vi "PicoScope4000ExampleAdvancedTrigger.vi"() -> ()   [LabVIEW 2012]
doc: "This example demonstrates how to use the PicoScope Labview library to collect data using block mode."
uses:
  shared/PicoBuffers.ctl
  shared/Acquisition Settings.ctl
  PicoScope4000Lib/PicoScope4000AnalogChannelSettingsIEPE.ctl
  PicoScope4000Lib/PicoScope4000Buffer and Transfer Settings.ctl
panel:
  in  "Pulse Width Qualifier Conditions":T1 {"Aux" items=["Don't Care", "True", "False"]; "Ext" items=["Don't Care", "True", "False"]; "Channel D" items=["Don't Care", "True", "False"]; "Channel C" items=["Don't Care", "True", "False"]; "Channel B" items=["Don't Care", "True", "False"]; "Channel A" items=["Don't Care", "True", "False"]; "Condition Logic" items=["AND", "OR", "XOR"]}
  in  "Trigger Conditions":T2 {"Aux" items=["Don't Care", "True", "False"]; "Pulse Width Qualifier" items=["Don't Care", "True", "False"]; "Ext" items=["Don't Care", "True", "False"]; "Channel D" items=["Don't Care", "True", "False"]; "Channel C" items=["Don't Care", "True", "False"]; "Channel B" items=["Don't Care", "True", "False"]; "Channel A" items=["Don't Care", "True", "False"]; "Condition Logic" items=["AND", "OR", "XOR"]}
  in  "Auto Trigger (ms)":i32=1000
  in  "Pulse Width Qualifier Settings":T3={"Direction"=2, "Lower Limit"=0, "Upper Limit"=0, "Pulse Width Type"=1} {"Pulse Width Type" items=["None", "Less Than", "Greater Than", "In Range", "Out of Range"]; "Direction" items=["Rising"=2, "Falling"=3, "Rising Lower"=7, "Above"=0, "Below"=1, "Rising or Falling"=4, "Falling Lower"=8, "Below Lower"=6, "Above Lower"=5]}
  in  "Channel Trigger Properties":T4={"Channel A Trigger Properties"={"thresholdUpper"=0, "thresholdUpperHysteresis"=0, "thresholdLower"=0, "thresholdLowerHysteresis"=0, "Threshold Mode"=0, "Direction"=2, "Available"=TRUE}, "Channel B Trigger Properties"={"thresholdUpper"=0, "thresholdUpperHysteresis"=0, "thresholdLower"=0, "thresholdLowerHysteresis"=0, "Threshold Mode"=0, "Direction"=2, "Available"=FALSE}, "Channel C Trigger Properties"={"thresholdUpper"=0, "thresholdUpperHysteresis"=0, "thresholdLower"=0, "thresholdLowerHysteresis"=0, "Threshold Mode"=0, "Direction"=2, "Available"=FALSE}, "Channel D Trigger Properties"={"thresholdUpper"=0, "thresholdUpperHysteresis"=0, "thresholdLower"=0, "thresholdLowerHysteresis"=0, "Threshold Mode"=0, "Direction"=2, "Available"=FALSE}} {"Channel D Trigger Properties"."Direction" items=["Above / Inside", "Below / Outside", "Rising / Enter", "Falling / Exit", "Rising or Falling / Enter or Exit", "Above Lower", "Below Lower", "Rising Lower", "Falling Lower", "Positive Runt", "Negative Runt"]; "Channel D Trigger Properties"."Threshold Mode" items=["Level", "Window"]; "Channel C Trigger Properties"."Direction" items=["Above / Inside", "Below / Outside", "Rising / Enter", "Falling / Exit", "Rising or Falling / Enter or Exit", "Above Lower", "Below Lower", "Rising Lower", "Falling Lower", "Positive Runt", "Negative Runt"]; "Channel C Trigger Properties"."Threshold Mode" items=["Level", "Window"]; "Channel B Trigger Properties"."Direction" items=["Above / Inside", "Below / Outside", "Rising / Enter", "Falling / Exit", "Rising or Falling / Enter or Exit", "Above Lower", "Below Lower", "Rising Lower", "Falling Lower", "Positive Runt", "Negative Runt"]; "Channel B Trigger Properties"."Threshold Mode" items=["Level", "Window"]; "Channel A Trigger Properties"."Direction" items=["Above / Inside", "Below / Outside", "Rising / Enter", "Falling / Exit", "Rising or Falling / Enter or Exit", "Above Lower", "Below Lower", "Rising Lower", "Falling Lower", "Positive Runt", "Negative Runt"]; "Channel A Trigger Properties"."Threshold Mode" items=["Level", "Window"]}
  in  "Channel B Settings":T5={"Enabled"=FALSE, "Range"=6, "Bandwidth Limit"=0, "Coupling"=1} {"Coupling" items=["AC", "DC", "IEPE"]; "Bandwidth Limit" items=["Off", "200kHz"]; "Range" items=["10 mV", "20 mV", "50 mV", "100 mV", "200 mV", "500 mV", "1 V", "2 V", "5 V", "10 V", "20 V", "50 V ", "100 V"]}
  out "Unit Info":T6
  in  "PS4262 Ext. Trigger Range":u32(ring)=5 items=["500 mV"=5, "5 V"=8]
  in  "Channel A Settings":T5={"Enabled"=TRUE, "Range"=6, "Bandwidth Limit"=0, "Coupling"=1} {"Coupling" items=["AC", "DC", "IEPE"]; "Bandwidth Limit" items=["Off", "200kHz"]; "Range" items=["10 mV", "20 mV", "50 mV", "100 mV", "200 mV", "500 mV", "1 V", "2 V", "5 V", "10 V", "20 V", "50 V ", "100 V"]}
  out "overflow":i16 format="%08b"
  in  "Apply Settings":bool
  out "error out":errorcluster
  in  "Data file":path=path "PicoScope4000ExampleBlock ChA Data"
  in  "Buffer and Transfer Settings":T7={"startIndex"=0, "Samples"=1000000, "Down Sample Ratio"=1, "Down-Sample Mode"=0} {"Down-Sample Mode" items=["None", "Aggregate", "Average"]; "Down Sample Ratio" step=1; "Samples" format="%_6p"}
  in  "Acquisition Settings":T8={"preTriggerSamples"=0, "postTriggerSamples"=1000000, "timebase"=3} {"postTriggerSamples" format="%_6p"; "preTriggerSamples" format="%_6p"}
  out "Properties Panel":T9 {"Max Total Capture Time Available (sec)" format="%.3p"; "Sample Frequency" format="%.6p"; "Sample Rate" format="%.3p"; "Max Samples Available" format="%_6p"; "Total Capture Time (sec)" format="%.3p"}
  in  "stop":bool
  out "Analog Channels":cluster{i32, dbl, "Data":dbl[]}[](graph)
  in  "Serial Number":string
  in  "Use Serial Number":bool
  in  "error in (no error)":errorcluster
  # "Bit 0 = ChA"
  # "For Condition Logic Suggested settings;\nFor AND, XOR logic-(parallel triggers)\nUse level-type triggers (Level or Inside/outside Window Triggers)\n\nFor OR logic- (single channel)\nUse edge types (e.g. rising, falling, entering window)"
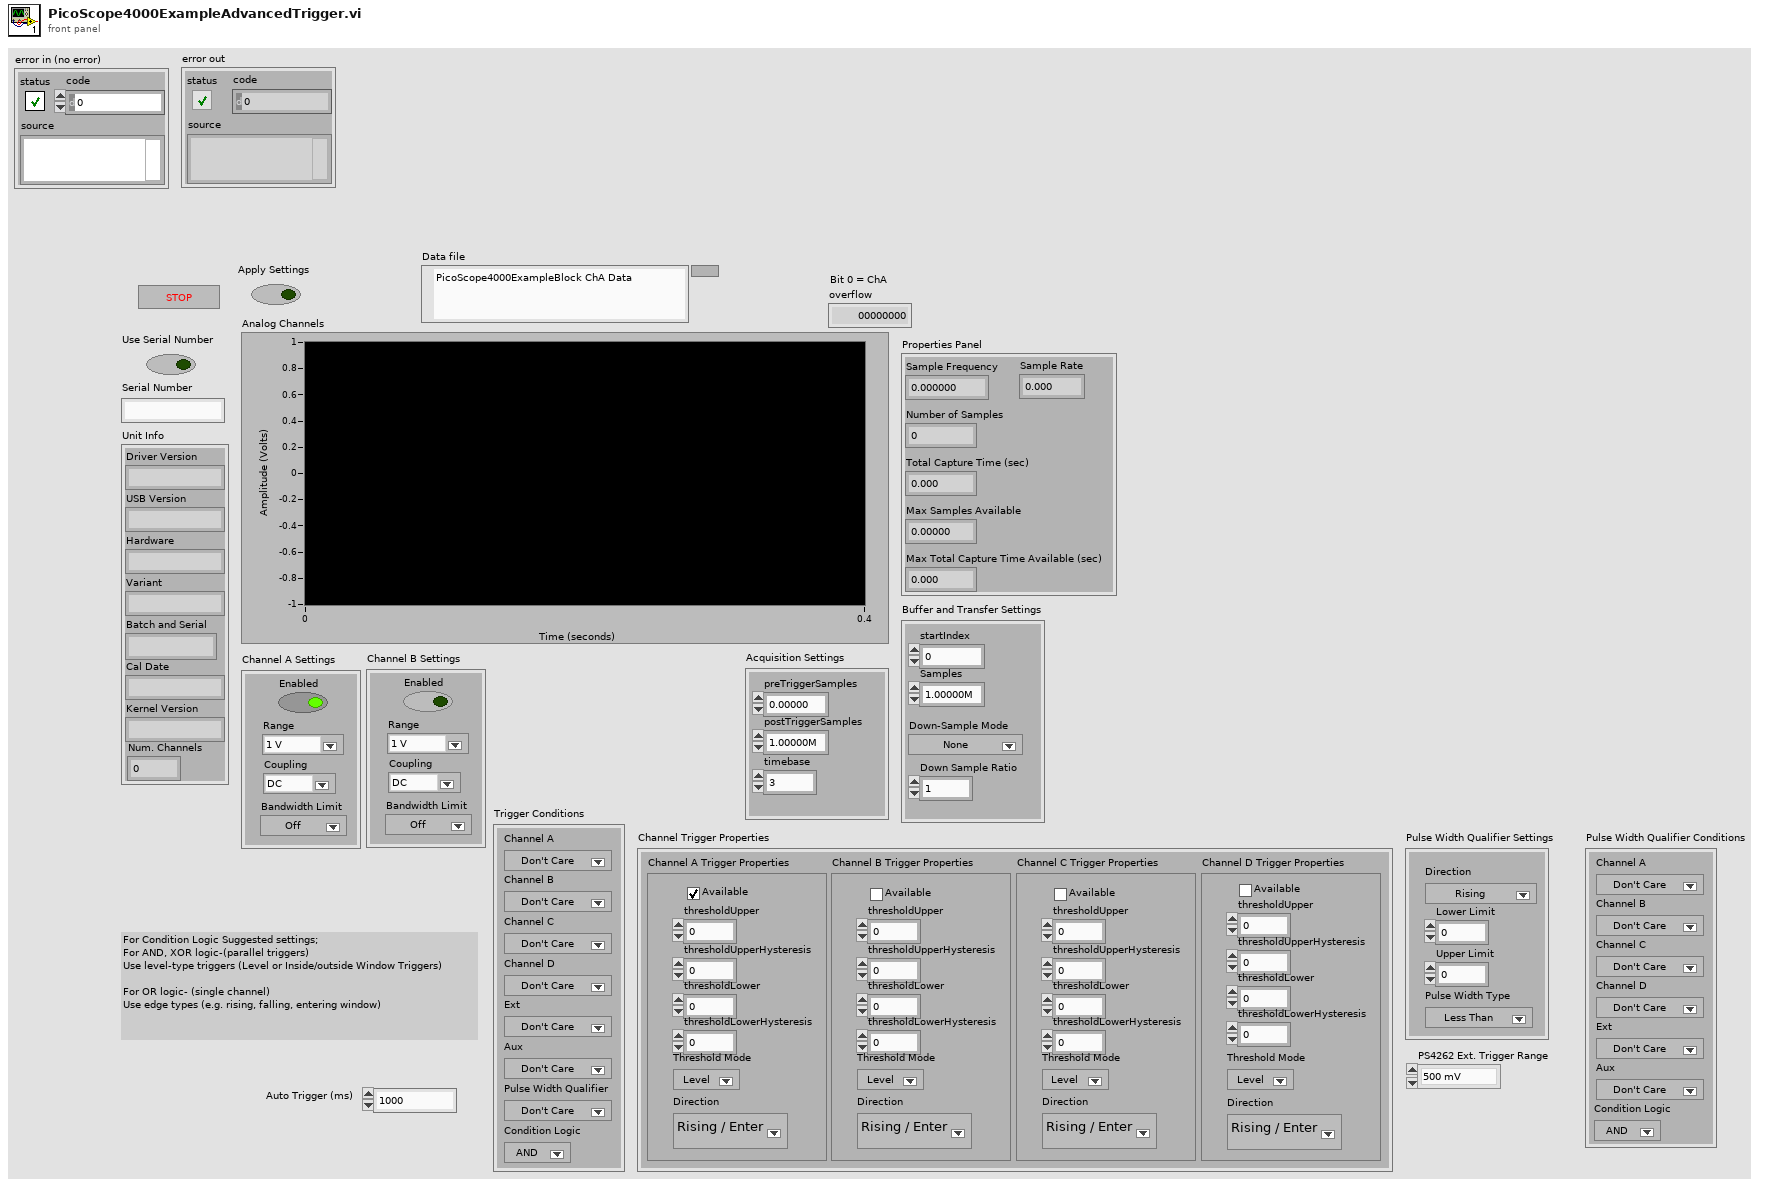
[diagram p1: front panel]
types:
  T1 = cluster{"Channel A":u16, "Channel B":u16, "Channel C":u16, "Channel D":u16, "Ext":u16, "Aux":u16, "Condition Logic":u16}
  T2 = cluster{"Channel A":u16, "Channel B":u16, "Channel C":u16, "Channel D":u16, "Ext":u16, "Aux":u16, "Pulse Width Qualifier":u16, "Condition Logic":u16}
  T3 = cluster{"Direction":u32, "Lower Limit":u32, "Upper Limit":u32, "Pulse Width Type":u32}
  T4 = cluster{"Channel A Trigger Properties":cluster{"thresholdUpper":i16, "thresholdUpperHysteresis":u16, "thresholdLower":i16, "thresholdLowerHysteresis":u16, "Threshold Mode":i32, "Direction":u32, "Available":bool}, "Channel B Trigger Properties":cluster{"thresholdUpper":i16, "thresholdUpperHysteresis":u16, "thresholdLower":i16, "thresholdLowerHysteresis":u16, "Threshold Mode":i32, "Direction":u32, "Available":bool}, "Channel C Trigger Properties":cluster{"thresholdUpper":i16, "thresholdUpperHysteresis":u16, "thresholdLower":i16, "thresholdLowerHysteresis":u16, "Threshold Mode":i32, "Direction":u32, "Available":bool}, "Channel D Trigger Properties":cluster{"thresholdUpper":i16, "thresholdUpperHysteresis":u16, "thresholdLower":i16, "thresholdLowerHysteresis":u16, "Threshold Mode":i32, "Direction":u32, "Available":bool}}
  T5 = typedef "PicoScope4000AnalogChannelSettingsIEPE.ctl" = cluster{"Enabled":bool, "Range":u16, "Bandwidth Limit":i16, "Coupling":u16}
  T6 = cluster{"Driver Version":string, "USB Version":string, "Hardware":string, "Variant":string, "Batch and Serial":string, "Cal Date":string, "Kernel Version":string, "Num. Channels":i16}
  T7 = typedef "PicoScope4000Buffer and Transfer Settings.ctl" = cluster{"startIndex":u64, "Samples":u64, "Down Sample Ratio":u64, "Down-Sample Mode":u32}
  T8 = typedef "Acquisition Settings.ctl" = cluster{"preTriggerSamples":u64, "postTriggerSamples":u64, "timebase":u32}
  T9 = cluster{"Sample Frequency":dbl, "Sample Rate":dbl, "Max Samples Available":u64, "Number of Samples":u64, "Total Capture Time (sec) ":dbl, "Max Total Capture Time Available (sec)":dbl}
  T10 = enum16{"open", "open or create", "create or replace", "create", "open (read-only)"}
  T11 = typedef "PicoBuffers.ctl" = cluster{"Max Buffer Pointers":u64[][][], "Min Buffer Pointers":u64[][][], "StreamingDataInfo":cluster{"Channel":u32, "Down-Sample Mode":u32, "PICO_DATA_TYPE":enum32{"PICO_INT8_T", "PICO_INT16_T", "PICO_INT32_T", "PICO_UINT32_T", "PICO_INT64_T", ""}, "Samples":i32, "bufferIndex":u64, "startIndex":i32, "overflow":i16}[][]}
  T12 = cluster{"Channel A Buffer":i16[], "Channel B Buffer":i16[], "Channel C Buffer":i16[], "Channel D Buffer":i16[], "Channel E Buffer":i16[], "Channel F Buffer":i16[], "Channel G Buffer":i16[], "Channel H Buffer":i16[], "Port 0 Buffer":i16[], "Port 1 Buffer":i16[]}[]
  T13 = cluster{"Channel A Buffer":i16[], "Channel B Buffer":i16[], "Channel C Buffer":i16[], "Channel D Buffer":i16[], "Channel E Buffer":i16[], "Channel F Buffer":i16[], "Channel G Buffer":i16[], "Channel H Buffer":i16[], "Port 0 Buffer":i16[], "Port 1 Buffer":i16[]}
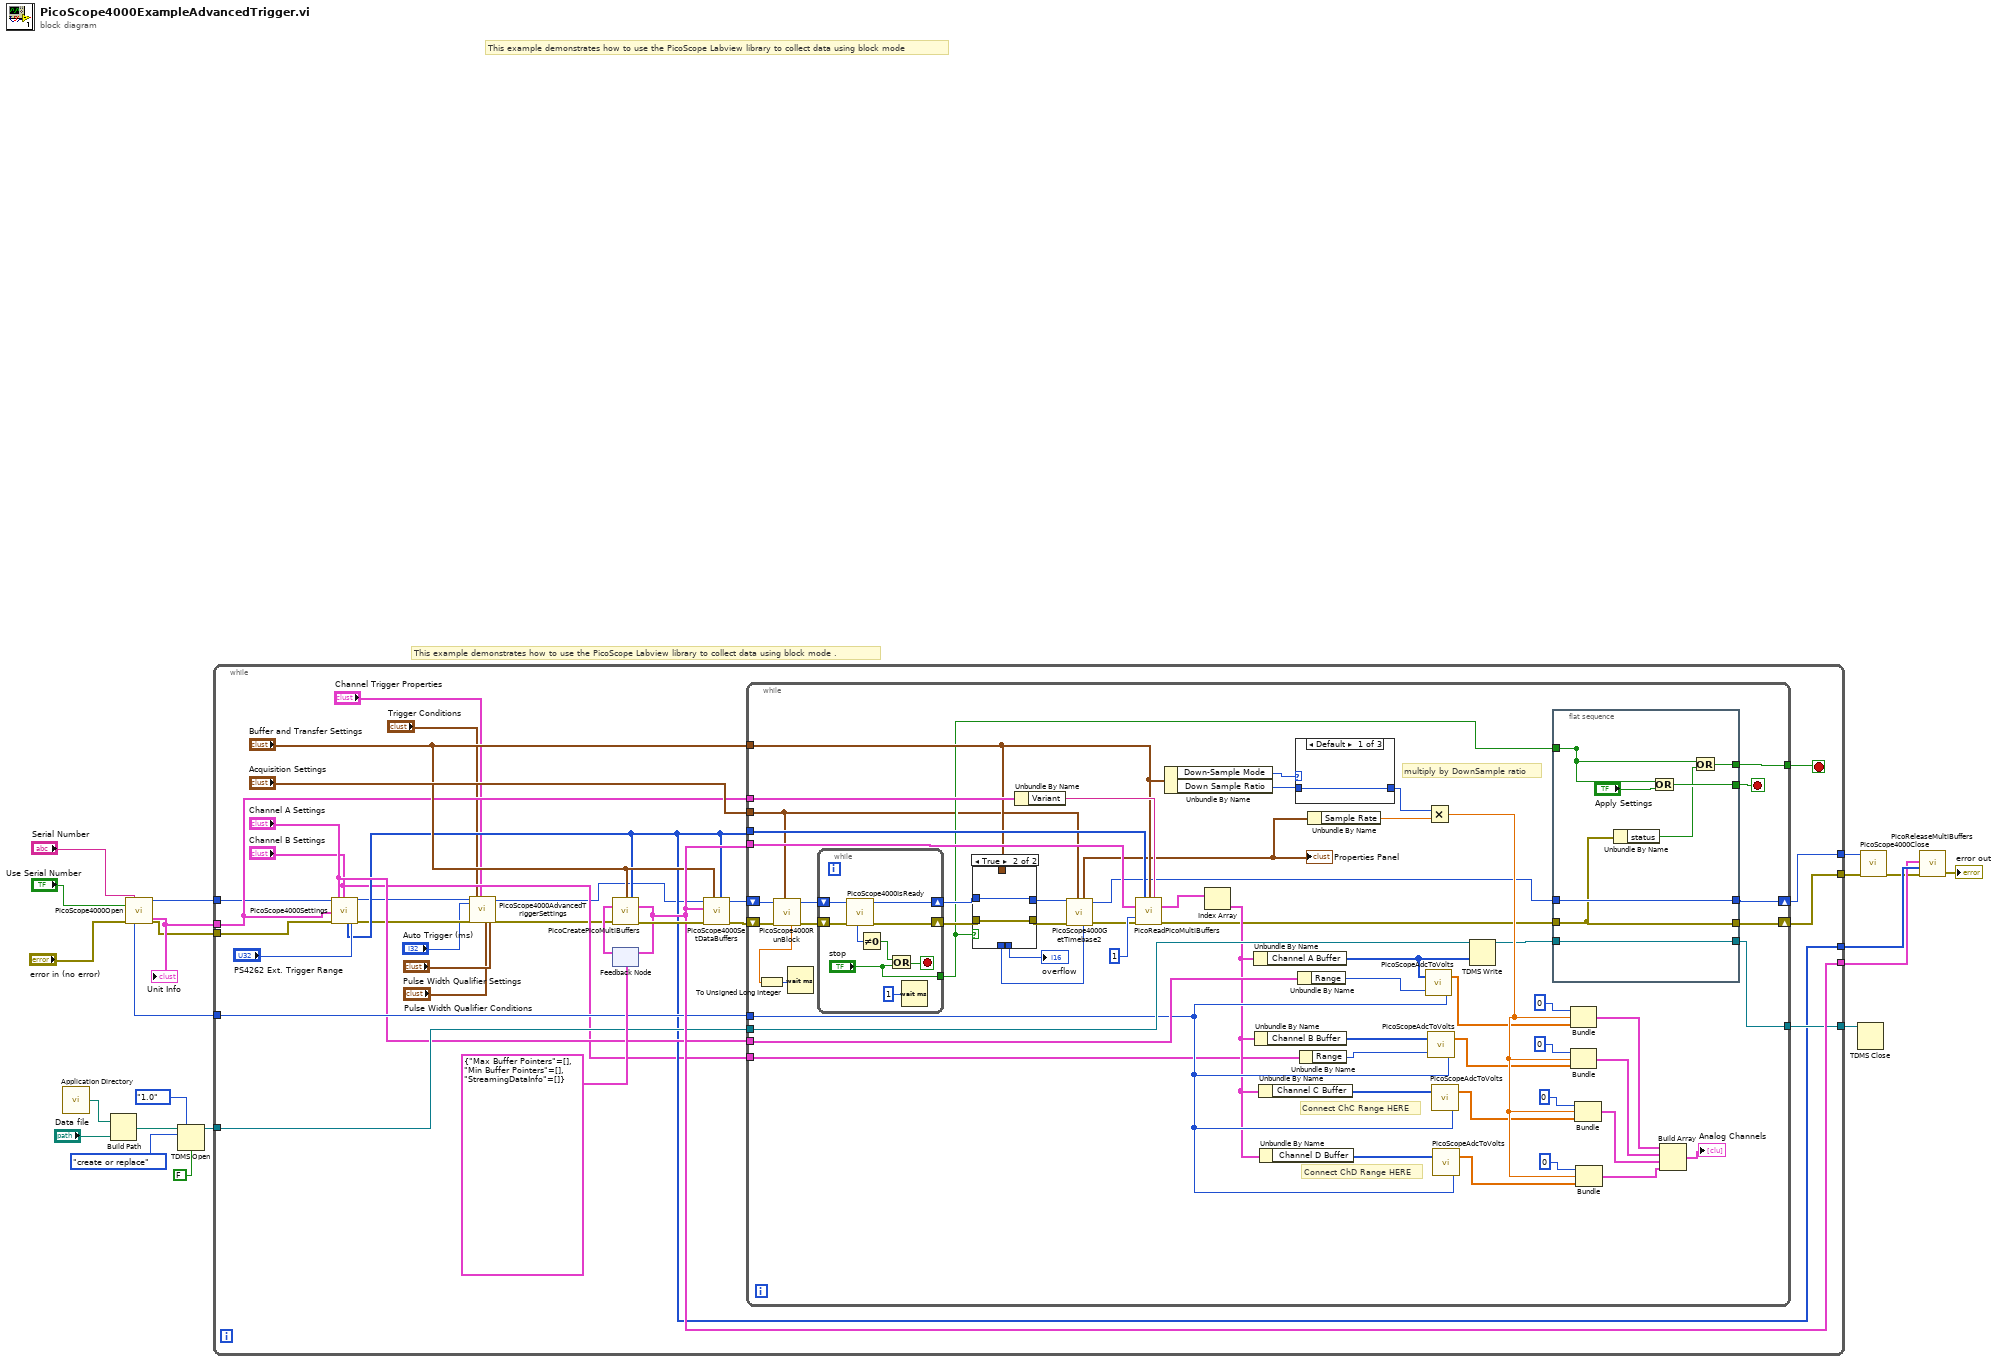
[diagram p0: block diagram]
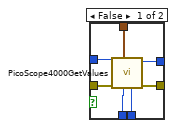
[diagram p2: hidden frame]
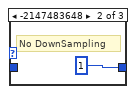
[diagram p3: hidden frame]
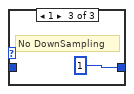
[diagram p4: hidden frame]
diagram:
  # "This example demonstrates how to use the PicoScope Labview library to collect data using block mode ."
  # "This example demonstrates how to use the PicoScope Labview library to collect data using block mode"
  n1 = call <vilib>:"Application Directory.vi"() -> ("Application Directory"=w14:path)
  n2 = Build Path(base path=w14, name or relative path="Data file") -> (appended path=w15:path)
  n3 = call "PicoScope4000Open.vi"("Serial Number"="Serial Number", "Use Serial Number"="Use Serial Number", "error in (no error)"="error in (no error)") -> ("handle"=w5:i16, "Max ADC value"=w10:i16, "Unit Info"=w6:T6, "error out"=w4:errorcluster)  [unwired: 9 in]
  "Unit Info" <- w6
  n4 = TDMS Open(6:FALSE ("disable buffering? (T)"), 7:enum16{"1.0", "2.0"}."1.0" ("file format version (2.0)"), 10:T10."create or replace" ("operation (0:open)"), 11:w15) -> (3:w12:refnum<k34>)  [unwired: 2 in, 1 out]
  n5 = while {
    tunnel: w10 -> [w45]
    tunnel: [w32] -> w21
    tunnel: [w48] -> w20
    tunnel: [w43] -> w13
    tunnel: w12 -> [w47]
    tunnel: [w44] -> w2
    tunnel: [w41] -> w9
    tunnel: w6 -> [w35]
    tunnel: w5 -> [w34]
    tunnel: w4 -> [w33]
    stop <- w42 stop-if-true
    n6 = call "PicoScope4000Settings.vi"("handle in"=w34, "Unit Info"=w35, "error in"=w33, "Channel A Settings"="Channel A Settings", "Channel B Settings"="Channel B Settings", "PicoScope 4262 Ext. Trigger Range"="PS4262 Ext. Trigger Range") -> ("Enabled array"=w32:i16[], "handle out"=w29:i16, "error out"=w30:errorcluster)  [unwired: 11 in]
    n7 = call "PicoScope4000AdvancedTriggerSettings.vi"("handle in"=w29, "error in"=w30, "Trigger Conditions"="Trigger Conditions", "Channel Trigger Properties"="Channel Trigger Properties", "Auto Trigger (ms)"="Auto Trigger (ms)", "Pulse Width Qualifier Conditions"="Pulse Width Qualifier Conditions", "Pulse Width Qualifier Settings"="Pulse Width Qualifier Settings") -> ("handle out"=w22:i16, "error out"=w23:errorcluster)  [unwired: 11 in]
    n8 = feedback #1(T11 {"Max Buffer Pointers"=[], "Min Buffer Pointers"=[], "StreamingDataInfo"=[]} ("Data Pointers")) -> (w50:T11)
    n9 = call "PicoCreatePicoMultiBuffers.vi"("Buffer and Transfer Settings"="Buffer and Transfer Settings", "enabled array"=w32, "Data Pointers In"=w50, "error in (no error)"=w23) -> ("Data Pointers"=w48:T11, "error out"=w49:errorcluster)  [unwired: 10 in]
    n10 = feedback-in #1(w48) -> ()
    n11 = call "PicoScope4000SetDataBuffers.vi"("enabled array"=w32, "Buffer and Transfer Settings"="Buffer and Transfer Settings", "error in (no error)"=w49, "Data Pointers In"=w48, "handle in"=w22) -> ("error out"=w40:errorcluster, "handle out"=w39:i16)  [unwired: 5 in]
    n12 = while {
      tunnel: w48 -> [w111]
      tunnel: "Buffer and Transfer Settings" -> [w65]
      tunnel: w32 -> [w102]
      tunnel: "Channel A Settings" -> [w101]
      tunnel: "Acquisition Settings" -> [w56]
      tunnel: w45 -> [w100]
      tunnel: w35 -> [w97]
      tunnel: [w72] -> w42
      shift-right: [w76] -> w44
      shift-left: w40 -> [w66]
      shift-right: [w70] -> w41
      shift-left: w39 -> [w67]
      tunnel: w47 -> [w110]
      tunnel: [w74] -> w43
      tunnel: "Channel B Settings" -> [w53]
      stop <- w71 stop-if-true
      # "Connect ChD Range HERE"
      # "Connect ChC Range HERE"
      # "multiply by DownSample ratio"
      n13 = call "PicoScope4000RunBlock.vi"("Acquisition Settings"=w56, "error in (no error)"=w66, "handle in"=w67) -> ("error out"=w104:errorcluster, "handle out"=w103:i16, "timeIndisposedMs"=w54:dbl)  [unwired: 5 in, 1 out]
      n14 = To Unsigned Long Integer(number=w54) -> (unsigned 32bit integer=w55:u32)
      n15 = Wait (ms)(milliseconds to wait=w55) -> ()  [unwired: 1 out]
      n16 = while {
        shift-right: [w136] -> w68
        shift-left: w104 -> [w137]
        shift-right: [w135] -> w69
        shift-left: w103 -> [w134]
        tunnel: ["stop"] -> w64
        stop <- w131 stop-if-true
        n17 = call "PicoScope4000IsReady.vi"("error in (no error)"=w137, "handle in"=w134) -> ("error out"=w136:errorcluster, "handle out"=w135:i16, "ready"=w133:i16)  [unwired: 7 in]
        n18 = Not Equal To 0?(x=w133) -> (x != 0?=w132:bool)
        n19 = Or(x=w132, y="stop") -> (x .or. y?=w131:bool)
        n20 = Wait (ms)(milliseconds to wait=u32 1) -> ()  [unwired: 1 out]
      }
      n21 = case shown="True" w64 {
        tunnel: w68 -> [w118 w119]
        tunnel: w69 -> [w117 w120]
        tunnel: [w116 w120] -> w58
        tunnel: [w115 w119] -> w59
        tunnel: w65 -> [w114 _]
        tunnel: [w113 _] -> w63
        tunnel: [w112 _] -> w62
        frame False {
          n22 = call "PicoScope4000GetValues.vi"("Buffer and Transfer Settings"=w114, "error in (no error)"=w118, "handle in"=w117) -> ("error out"=w115:errorcluster, "handle out"=w116:i16, "overflow"=w113:i16, "noOfSamples"=w112:u64)  [unwired: 5 in]
        }
        frame True {
        }
      }
      "overflow" <- w63
      n23 = Unbundle By Name(w97) -> ("Variant"=w98:string)
      n24 = call "PicoScope4000GetTimebase2.vi"("Number of Samples"=w62, "Acquisition Settings"=w56, "error in (no error)"=w59, "handle in"=w58) -> ("error out"=w60:errorcluster, "handle out"=w57:i16, "Properties Panel"=w61:T9)  [unwired: 5 in]
      "Properties Panel" <- w61
      n25 = call "PicoReadPicoMultiBuffers.vi"("enabled array"=w102, "Buffer and Transfer Settings"=w65, "Variant"=w98, "Data Pointers"=w111, "No of Buffers"=1, "error in (no error)"=w60) -> ("MultiBuffers (Max or non-aggregated)"=w109:T12, "error out"=w73:errorcluster)  [unwired: 7 in, 1 out]
      n26 = Unbundle By Name(w65) -> ("Down-Sample Mode"=w107:u32, "Down Sample Ratio"=w108:u64)
      n27 = Index Array(array=w109) -> (element=w77:T13)  [unwired: 1 in]
      n28 = Unbundle By Name(w77) -> ("Channel A Buffer"=w86:i16[])
      n29 = Unbundle By Name(w77) -> ("Channel B Buffer"=w92:i16[])
      n30 = Unbundle By Name(w77) -> ("Channel C Buffer"=w84:i16[])
      n31 = Unbundle By Name(w77) -> ("Channel D Buffer"=w80:i16[])
      n32 = case shown="Default" w107 {
        tunnel: [w138 u64 1 ("Down Sample Ratio") u64 1 ("Down Sample Ratio")] -> w105
        tunnel: w108 -> [w138 _ _]
        frame Default {
        }
        frame -2147483648 {
          # "No DownSampling"
        }
        frame 1 {
          # "No DownSampling"
        }
      }
      n33 = Unbundle By Name(w101) -> ("Range"=w94:u16)
      n34 = Unbundle By Name(w53) -> ("Range"=w52:u16)
      n35 = Unbundle By Name(w61) -> ("Sample Rate"=w99:dbl)
      n36 = call "PicoScopeAdcToVolts.vi"("Max_adc"=w100, "Range Index"=w94, "Data"=w86) -> ("Data"=w87:dbl[])
      n37 = Multiply(x=w105, y=w99) -> (x*y=w106:dbl)
      n38 = call "PicoScopeAdcToVolts.vi"("Max_adc"=w100, "Range Index"=w52, "Data"=w92) -> ("Data"=w91:dbl[])
      n39 = call "PicoScopeAdcToVolts.vi"("Max_adc"=w100, "Data"=w84) -> ("Data"=w83:dbl[])  [unwired: 1 in]
      n40 = call "PicoScopeAdcToVolts.vi"("Max_adc"=w100, "Data"=w80) -> ("Data"=w79:dbl[])  [unwired: 1 in]
      n41 = TDMS Write(0:w110, 9:w86) -> (4:w75:refnum<k34>)  [unwired: 4 in, 3 out]
      n42 = flat-sequence {
        tunnel: [w128] -> w71
        tunnel: [w121] -> _
        tunnel: [w125] -> w72
        tunnel: w57 -> [w124]
        tunnel: [w124] -> w70
        tunnel: w73 -> [w123]
        tunnel: [w123] -> w76
        tunnel: [w122] -> w74
        tunnel: w75 -> [w122]
        tunnel: w64 -> [w121]
        frame #0 {
          n43 = Unbundle By Name(w123) -> ("status"=w126:bool)
          n44 = Or(x=w121, y="Apply Settings") -> (x .or. y?=w128:bool)
          n45 = Or(x=w121, y=w126) -> (x .or. y?=w125:bool)
        }
      }
      n46 = Bundle(0, w106, "Data"=w87) -> (w90:cluster{i32, dbl, "Data":dbl[]})  [unwired: 1 in]
      n47 = Bundle(0, w106, "Data"=w91) -> (w89:cluster{i32, dbl, "Data":dbl[]})  [unwired: 1 in]
      n48 = Bundle(0, w106, "Data"=w83) -> (w82:cluster{i32, dbl, "Data":dbl[]})  [unwired: 1 in]
      n49 = Bundle(0, w106, "Data"=w79) -> (w78:cluster{i32, dbl, "Data":dbl[]})  [unwired: 1 in]
      n50 = Build Array(w90, w89, w82, w78) -> (→"Analog Channels":cluster{i32, dbl, "Data":dbl[]}[])
    }
  }
  n51 = TDMS Close(11:w13) -> ()  [unwired: 1 in, 2 out]
  n52 = call "PicoScope4000Close.vi"("error in (no error)"=w2, "handle"=w9) -> ("error out"=w1:errorcluster)  [unwired: 9 in]
  n53 = call "PicoReleaseMultiBuffers.vi"("error in (no error)"=w1, "Enabled array"=w21, "Data Pointers"=w20) -> ("error out"=→"error out":errorcluster)  [unwired: 8 in]
